vi "ORS_AlazarDLLAcq_Prepare.vi"(5 "Lamda Trigger?":bool, 6 "Channel":u32(ring)=1 items=["A"=1, "B"=2, "A + B"=3, "C"=4, "A + C"=5, "A + B"=6, "D"=8, "A + D"=9, "B + D"=10, "C + D"=12, "A + B + C + D"=15], 7 "Records Per Buffer":u32=1000, 8 "error in (no error)":errorcluster, 9 "Records Count":u32=2000, 10 "Record length":u32=2048, 11 "ATSHandle":u32) -> (0 "error out":errorcluster, 2 "Samps Per Buffer":u32, 3 "ATSHandle_out":u32)   [LabVIEW 2024]
panel:
  out "Return Code":u32
  in  "free mem?":bool
  in  "channel":enum16{"A", "B", "A & B"}(ring)
  in  "record_len":u32=8192
  out "path out":path
  out "return code":i32
  out "dt":u32=26
  in  "n_records":u32=1
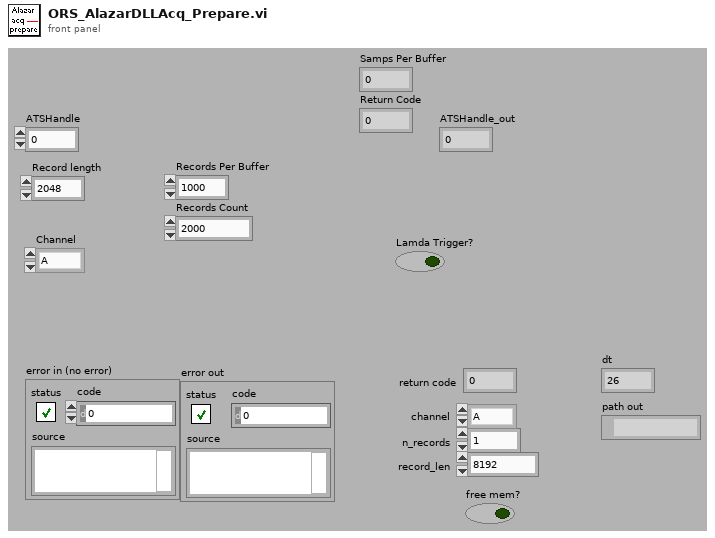
[diagram p1: front panel]
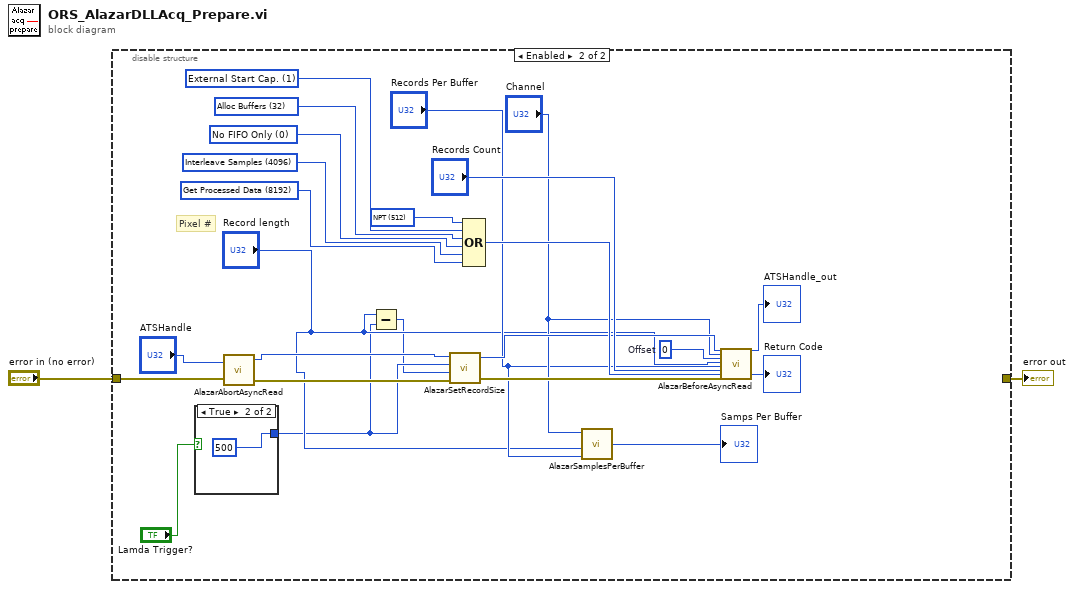
[diagram p0: block diagram]
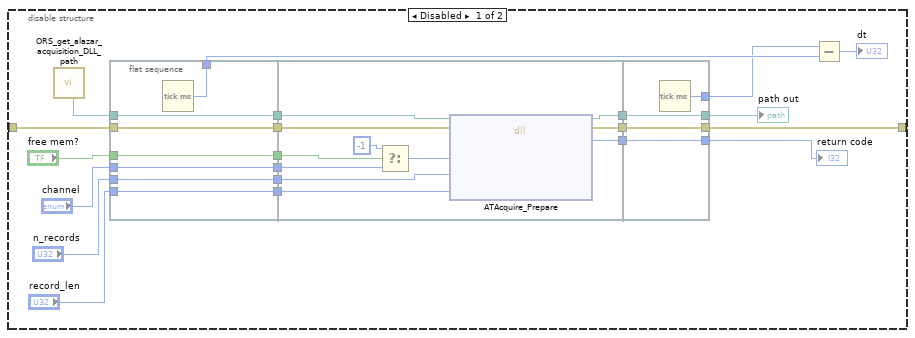
[diagram p2: hidden frame]
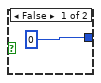
[diagram p3: hidden frame]
diagram:
  n1 = disable-structure shown="Enabled" {
    disable-tunnel: "error in (no error)" -> [w4 w54]
    disable-tunnel: [w3 _] -> w1
    frame Disabled {
      n2 = call "ORS_get_alazar_acquisition_DLL_path.vi"() -> ("Alazar Acquisition DLL path"=w5:path)  [unwired: 10 in, 1 out]
      n3 = flat-sequence {
        tunnel: w5 -> [w29]
        tunnel: "n_records" -> [w30]
        tunnel: [w30] -> w23
        tunnel: [w29] -> w22
        tunnel: [w28] -> w12
        tunnel: "channel" -> [w27]
        tunnel: [w27] -> w21
        tunnel: [w26] -> w20
        tunnel: "record_len" -> [w26]
        tunnel: [w25] -> w19
        tunnel: "free mem?" -> [w25]
        tunnel: w4 -> [w24]
        tunnel: [w24] -> w18
        tunnel: [w41] -> w17
        tunnel: w23 -> [w40]
        tunnel: w22 -> [w39]
        tunnel: [w38] -> w16
        tunnel: w21 -> [w33]
        tunnel: w20 -> [w37]
        tunnel: w19 -> [w36]
        tunnel: [w32] -> w15
        tunnel: w18 -> [w31]
        tunnel: [w45] -> w13
        tunnel: w17 -> [w45]
        tunnel: [w44] -> w11
        tunnel: [w43] -> w9
        tunnel: w16 -> [w43]
        tunnel: [w42] -> w3
        tunnel: w15 -> [w42]
        frame #0 {
          n4 = Tick Count (ms)() -> (millisecond timer value=w28:u32)
        }
        frame #1 {
          n5 = Select(t=-1, s=w36, f=w33) -> (s? t:f=w34:i32)
          n6 = dll-call lib="Z:/Software/AlazarTech/ATS-SDK/5.6.3/ATS9462-SDK/Dual Port Async/C/PostBuffer_Recommended/at_acquire/Release/at_acquire.dll" fn="ATAcquire_Prepare" ("at_acquire.dll:TestFunc")(path in=w39, error in=w31, "channel"=w34, "n_records"=w40, "record_len"=w37) -> (path out=w38:path, error out=w32:errorcluster, "return type"=w41:i32)  [unwired: 4 in]
        }
        frame #2 {
          n7 = Tick Count (ms)() -> (millisecond timer value=w44:u32)
        }
      }
      n8 = Subtract(x=w11, y=w12) -> (x-y=→"dt":u32)
      "return code" <- w13
      "path out" <- w9
    }
    frame Enabled {
      w68 = u32 0  # Offset
      w61 = u32 8192 items=["No Get Processed Data"=32, "Get Processed Data"=8192]
      w62 = u32 4096 items=["Not Interleaved Samples"=0, "Interleave Samples"=4096]
      w66 = u32 0 items=["No FIFO Only"=0, "FIFO Only"=2048]
      w63 = u32 32 items=["Alloc Buffers"=32]
      w64 = u32 1 items=["Internal Start Cap.", "External Start Cap."]
      w65 = u32 512 items=["Traditional"=0, "NPT"=512, "Continuous"=256, "Triggered Streaming"=1024]
      # "Pixel #"
      n9 = case shown="True" "Lamda Trigger?" {
        tunnel: [u32 0 ("Pre-trigger Samples") u32 500 ("Pre-trigger Samples")] -> w48
        frame False {
        }
        frame True {
        }
      }
      n10 = call "AlazarAbortAsyncRead.vi"("Handle"="ATSHandle", "error in (no error)"=w54) -> ("Handle"=w50:u32, "error out"=w53:errorcluster)  [unwired: 1 out]
      n11 = Subtract(x="Record length", y=w48) -> (x-y=w47:u32)
      n12 = call "AlazarSetRecordSize.vi"("error in (no error)"=w53, "Post-trigger Samples"=w47, "Pre-trigger Samples"=w48, "Handle"=w50) -> ("error out"=w59:errorcluster, "Handle"=w60:u32)  [unwired: 1 out]
      n13 = Compound Arithmetic op=OR(w65, w64, w63, w66, w62, w61) -> (w67:u32)
      n14 = call "AlazarSamplesPerBuffer.vi"("Records Per Buffer"="Records Per Buffer", "Samples Per Record"="Record length", "Channel Mask"="Channel") -> ("Samples Per Buffer"=→"Samps Per Buffer":u32)  [unwired: 1 in]
      n15 = call "AlazarBeforeAsyncRead.vi"("Handle"=w60, "Channel"="Channel", "Offset"=w68, "Length"="Record length", "Records Per Buffer"="Records Per Buffer", "Records Count"="Records Count", "cFlags"=w67, "error in (no error)"=w59) -> ("Handle"=→"ATSHandle_out":u32, "Return Code"=→"Return Code":u32)  [unwired: 17 in, 1 out]
    }
  }
  "error out" <- w1
